vi "mod_Modulate AM (VSB).vi"(0 "message signal":waveform(dbl), 2 "pilot tone":T1={"frequency (Hz)"=0.0, "amplitude"=1.0}, 5 "AM SSB-VSB parameters":T3={"modulation index"=1.0, "side-band"=enum."Lower sideband", "suppress carrier ?"=FALSE} {"modulation index" format="%.2f"}, 7 "VSB FIR filter design":T2={"#taps"=161, "lower PB (Hz)"=-0.0375, "upper PB (Hz)"=0.2, "lower SB (Hz)"=-0.0625, "upper SB (Hz)"=0.225} {"lower SB (Hz)" format="%0.2p"; "upper SB (Hz)" format="%0.2p"; "lower PB (Hz)" format="%0.2p"; "upper PB (Hz)" format="%0.2p"}, 9 "peak message amplitude":dbl=1.0, 11 "error in (no error)":errorcluster, 13 "reset? (T)":bool=TRUE) -> (4 "output complex waveform":T4={"t0"=0.0, "dt"=1.0, "Y"=[]} {"Y" format="%.3f"; "dt" format="%^.2e"; "t0" format="%.4f"}, 15 "error out":errorcluster)   [LabVIEW 2020, in "niAMT.lvlib"]
uses:
  <vilib>/addons/Modulation/niAMT.lvlib
  <vilib>/addons/Modulation/Analog/controls/Complex Data Waveform.ctl
  <vilib>/addons/Modulation/Analog/controls/mod_AM parameters.ctl
  <vilib>/addons/Modulation/Analog/controls/mod_AM VSB filter.ctl
  <vilib>/addons/Modulation/Analog/controls/mod_AM pilot tone.ctl
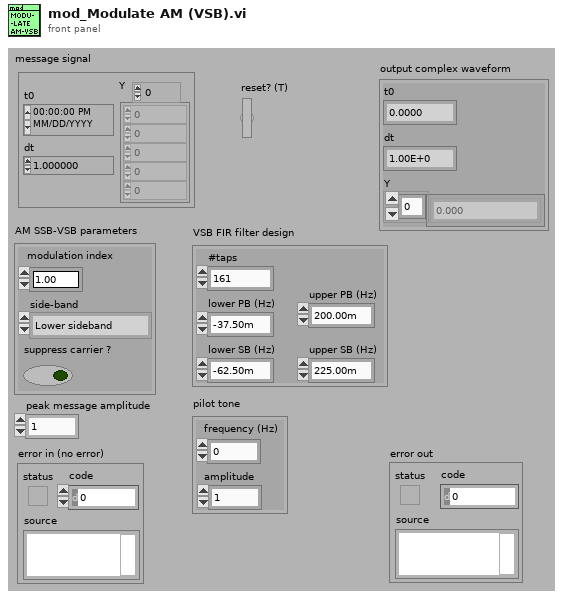
[diagram p1: front panel]
types:
  T1 = typedef "niAMT.lvlib/mod_AM pilot tone.ctl" = cluster{"frequency (Hz)":dbl, "amplitude":dbl}
  T2 = typedef "niAMT.lvlib/mod_AM VSB filter.ctl" = cluster{"#taps":i32, "lower PB (Hz)":dbl, "upper PB (Hz)":dbl, "lower SB (Hz)":dbl, "upper SB (Hz)":dbl}
  T3 = typedef "niAMT.lvlib/mod_AM parameters.ctl" = cluster{"modulation index":dbl, "side-band":enum16{"Lower sideband", "Upper sideband"}, "suppress carrier ?":bool}
  T4 = typedef "niAMT.lvlib/Complex Data Waveform.ctl" = cluster{"t0":dbl, "dt":dbl, "Y":cdb[]}
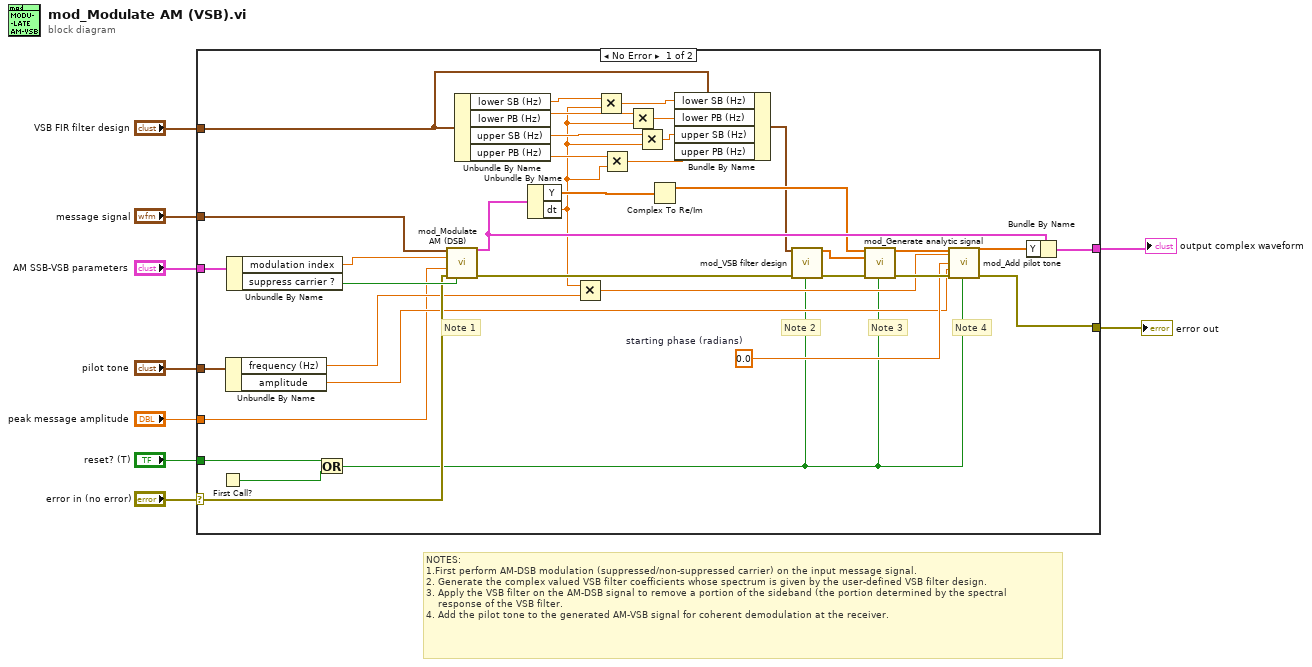
[diagram p0: block diagram]
diagram:
  # "NOTES:\n1.First perform AM-DSB modulation (suppressed/non-suppressed carrier) on the input message signal.\n2. Generate the complex valued VSB filter coefficients whose spectrum is given by the user-defined VSB filter design.\n3. Apply the VSB filter on the AM-DSB signal to remove a portion of the sideband (the portion determined by the spectral\n    response of the VSB filter.\n4. Add the pilot tone to the generated AM-VSB signal for coherent demodulation at the receiver."
  n1 = case shown="No Error" "error in (no error)" {
    selector: "error in (no error)" -> [w27 w46]
    tunnel: [w40 w46] -> w8
    tunnel: [w37 _] -> w7
    tunnel: "AM SSB-VSB parameters" -> [w29 _]
    tunnel: "message signal" -> [w28 _]
    tunnel: "reset? (T)" -> [w26 _]
    tunnel: "VSB FIR filter design" -> [w20 _]
    tunnel: "pilot tone" -> [w14 _]
    tunnel: "peak message amplitude" -> [w10 _]
    frame No Error {
      w36 = 0.0  # starting phase (radians)
      # "Note 4"
      # "Note 3"
      # "Note 2"
      # "Note 1"
      n2 = First Call?() -> (First Call?: T/F=w35:bool)
      n3 = Unbundle By Name(w14) -> ("frequency (Hz)"=w13:dbl, "amplitude"=w12:dbl)
      n4 = Unbundle By Name(w29) -> ("modulation index"=w31:dbl, "suppress carrier ?"=w30:bool)
      n5 = Or(x=w26, y=w35) -> (x .or. y?=w11:bool)
      n6 = call <vilib>:"mod_Modulate AM (DSB).vi"("message signal"=w28, "modulation index"=w31, "peak message amplitude"=w10, "error in (no error)"=w27, "suppress carrier ?"=w30) -> ("AM modulated waveform"=w45:cluster{"t0":dbl, "dt":dbl, "Y":cdb[]}, "error out"=w33:errorcluster)  [unwired: 2 in, 7 out]
      n7 = Unbundle By Name(w20) -> ("lower SB (Hz)"=w25:dbl, "lower PB (Hz)"=w24:dbl, "upper SB (Hz)"=w23:dbl, "upper PB (Hz)"=w22:dbl)
      n8 = Unbundle By Name(w45) -> ("Y"=w44:cdb[], "dt"=w21:dbl)
      n9 = Multiply(x=w21, y=w13) -> (x*y=w38:dbl)
      n10 = Multiply(x=w25, y=w21) -> (x*y=w19:dbl)
      n11 = Multiply(x=w22, y=w21) -> (x*y=w16:dbl)
      n12 = Multiply(x=w24, y=w21) -> (x*y=w18:dbl)
      n13 = Multiply(x=w23, y=w21) -> (x*y=w17:dbl)
      n14 = Complex To Re/Im(x + iy=w44) -> (x=w43:dbl[])  [unwired: 1 out]
      n15 = Bundle By Name(cluster=w20, "lower SB (Hz)"=w19, "lower PB (Hz)"=w18, "upper SB (Hz)"=w17, "upper PB (Hz)"=w16) -> (w15:T2)
      n16 = call <vilib>:"mod_VSB filter design.vi"("VSB FIR filter design"=w15, "error in (no error)"=w33, "reset ? (T)"=w11) -> ("VSB filter taps"=w34:cdb[], "error out"=w32:errorcluster)  [unwired: 3 in, 8 out]
      n17 = call <vilib>:"mod_Generate analytic signal.vi"("m(t)"=w43, "filter taps"=w34, "error in (no error)"=w32, "reset? (T)"=w11) -> ("analytic signal"=w42:cdb[], "error out"=w41:errorcluster)  [unwired: 10 out]
      n18 = call <vilib>:"mod_Add pilot tone.vi"("input"=w42, "pilot tone frequency (normalized)"=w38, "starting phase (radians)"=w36, "pilot tone amplitude"=w12, "error in (no error)"=w41, "reset? (T)"=w11) -> ("input+pilot tone"=w39:cdb[], "error out"=w40:errorcluster)  [unwired: 8 out]
      n19 = Bundle By Name(cluster=w45, "Y"=w39) -> (w37:cluster{"t0":dbl, "dt":dbl, "Y":cdb[]})
    }
    frame Error {
    }
  }
  "error out" <- w8
  "output complex waveform" <- w7
